vi "2_Match pattern.vi"() -> ()   [LabVIEW 2010]
uses:
  <vilib>/regexp/Match Regular Expression.xnode
panel:
  out "after match":string
  out "whole match":string
  out "before match":string
  out "after substring":string
  out "match substring":string
  out "before substring":string
  out "result string 2":string
  out "replaced substring":string
  out "result string":string
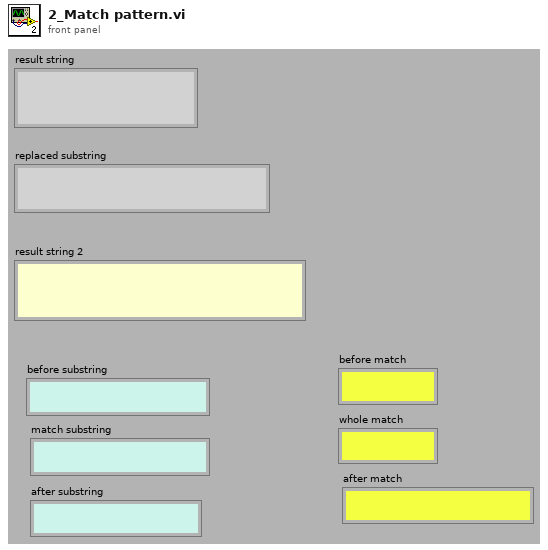
[diagram p1: front panel]
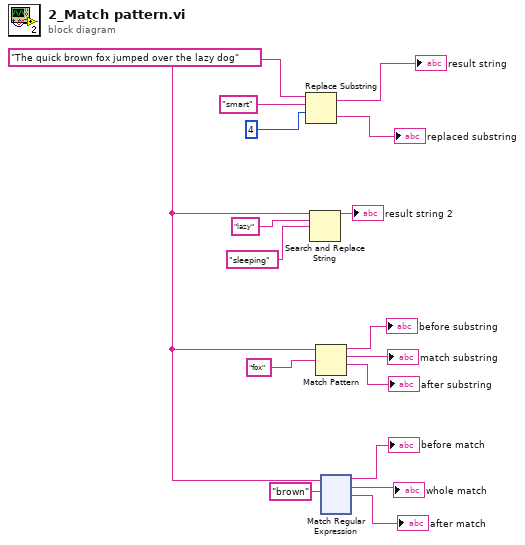
[diagram p0: block diagram]
diagram:
  w5 = "The quick brown fox jumped over the lazy dog" ("string")
  n1 = Replace Substring(3:4 ("offset (0)"), 4:"smart" ("substring (\"\")"), 5:w5) -> (0:→"replaced substring":string, 1:→"result string":string)  [unwired: 1 in]
  n2 = Search and Replace String(input string=w5, search string="lazy", replace string="sleeping" ("replace string (\"\")")) -> (result string=→"result string 2":string)  [unwired: 5 in, 3 out]
  n3 = Match Pattern(string=w5, regular expression="fox") -> (before substring=→"before substring":string, match substring=→"match substring":string, after substring=→"after substring":string)  [unwired: 1 in, 1 out]
  n4 = xnode "Match Regular Expression"("input string"=w5, "regular expression"="brown") -> ("before match"=→"before match":string, "whole match"=→"whole match":string, "after match"=→"after match":string)  [unwired: 4 in, 2 out]
